vi "ZMC Check Program Syntax.vi"(8 "error in (no error)":errorcluster caption="错误输入（无错误）", 10 "sError":string, 11 "pzpjfilename":string) -> (0 "error out":errorcluster caption="错误输出", 2 "sError out":string, 3 "function return":i32)   [LabVIEW 2015, in "zauxdll.lvlib"]
doc: "int32 __stdcall ZMC_CheckProgramSyntax(const char *pzpjfilename, char *sError);"
uses:
  zauxdll.lvlib
  zmotion.dll
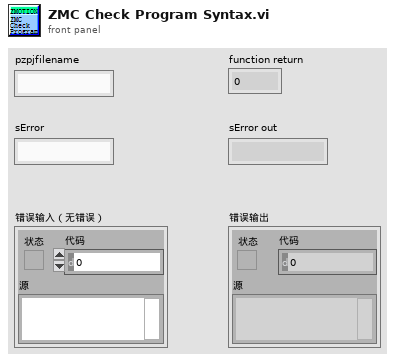
[diagram p1: front panel]
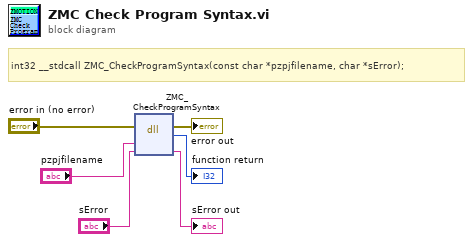
[diagram p0: block diagram]
diagram:
  # "int32 __stdcall ZMC_CheckProgramSyntax(const char *pzpjfilename, char *sError);"
  n1 = dll-call lib="C:/Users/VIC/Desktop/GOGORO_SA/system/LLB/zmotion/zaux/zmotion.*" fn="ZMC_CheckProgramSyntax"(error in="error in (no error)", "pzpjfilename"="pzpjfilename", "sError"="sError") -> (error out=→"error out":errorcluster, →"function return":i32, "sError"=→"sError out":string)  [unwired: 3 in, 1 out]
